vi "1 Channel N Samples - Manual Timestamps.vi"() -> ()   [LabVIEW 2026, in "synnax_lib.lvlib"]
uses:
  lvproj/lvlib/synnax_lib.lvlib
  lvproj/lvlib/typedefs/connection_config.ctl
  lvproj/lvlib/classes/Client/Private/synnax channel retrieve keys Single.vi
  lvproj/lvlib/classes/Writer/Private/synnax writer open Array.vi
  lvproj/lvlib/classes/Writer/Private/Writes/DBL/Write 1Ch NSamp (DBL).vi
  lvproj/lvlib/classes/Synnax Writer.lvclass
  lvproj/lvlib/classes/Client/Synnax Client.lvclass
panel:
  out "error out":errorcluster
  in  "Channel":string="my_f64_chan"
  in  "Stop":bool
  in  "Connection Config":T1={"host"="localhost", "port"=9090, "username"="synnax", "password"="seldon"}
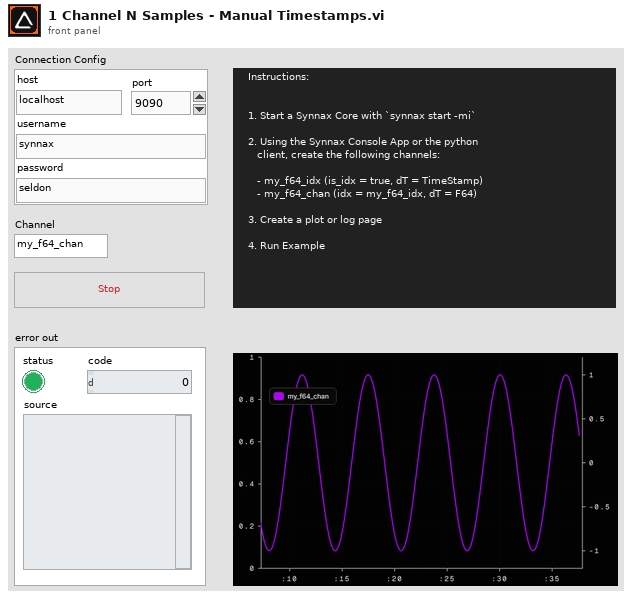
[diagram p1: front panel]
types:
  T1 = typedef "synnax_lib.lvlib/connection_config.ctl" = cluster{"host":string, "port":u16, "username":string, "password":string}
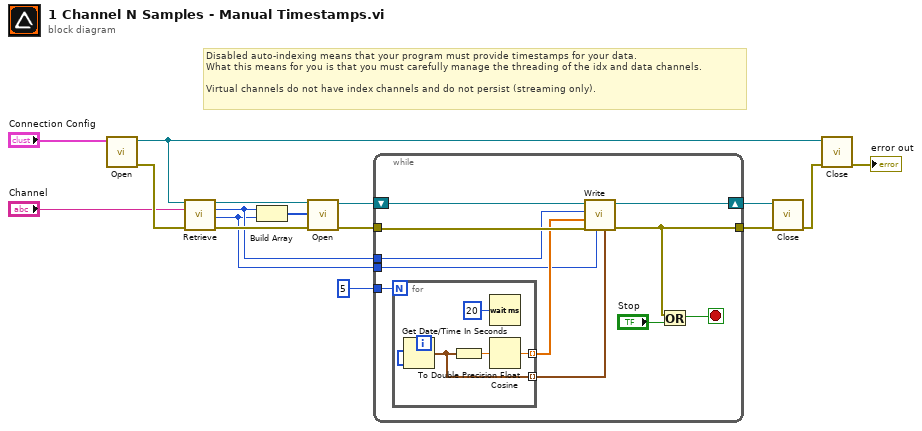
[diagram p0: block diagram]
diagram:
  # "Disabled auto-indexing means that your program must provide timestamps for your data.\nWhat this means for you is that you must carefully manage the threading of the idx and data channels.\n\nVirtual channels do not have index channels and do not persist (streaming only)."
  n1 = call "Open.vi"("Connection Config"="Connection Config") -> ("error out"=w11:errorcluster, "Synnax Client out"=w13:refnum<class "Synnax Client.lvclass">)  [unwired: 9 in]
  n2 = call-poly "Retrieve.vi"("Synnax Client in"=w13, "channel name"="Channel", "error in"=w11) -> ("Synnax Client out"=w7:refnum<class "Synnax Client.lvclass">, "channel key"=w4:u32, "index key"=w3:u32, "error out"=w15:errorcluster)  [unwired: 8 in, 1 out]
  n3 = Build Array(w4, w3) -> (w5:u32[])
  n4 = call-poly "Open.vi"("error in"=w15, "channels in"=w5, "Synnax Client in"=w7) -> ("error out"=w8:errorcluster, "writer out"=w10:refnum<class "Synnax Writer.lvclass">)  [unwired: 6 in, 1 out]
  n5 = while {
    shift-right: [w26] -> w9
    shift-left: w10 -> [w27]
    tunnel: w8 -> [w25]
    tunnel: [w17] -> w16
    tunnel: w3 -> [w22]
    tunnel: w4 -> [w20]
    tunnel: 5 -> [w19]
    stop <- w18 stop-if-true
    n6 = for {
      N: w19 -> [_]
      tunnel: [w31] -> w23 mode=indexing
      tunnel: [w29] -> w21 mode=indexing
      n7 = Get Date/Time In Seconds() -> (seconds since 1Jan1904=w29:timestamp)
      n8 = To Double Precision Float(number=w29) -> (double precision float=w30:dbl)
      n9 = Wait (ms)(milliseconds to wait=u32 20) -> ()  [unwired: 1 out]
      n10 = Cosine(x=w30) -> (cos(x)=w31:dbl)
    }
    n11 = call-poly "Write.vi"("timestamps"=w21, "index_channel"=w22, "error in"=w25, "data"=w23, "channel"=w20, "Writer"=w27) -> ("error out"=w17:errorcluster, "Writer Out"=w26:refnum<class "Synnax Writer.lvclass">)  [unwired: 4 in]
    n12 = Or(x=w17, y="Stop") -> (x .or. y?=w18:bool)
  }
  n13 = call "Close.vi"("error in"=w16, "writer"=w9) -> ("error out"=w12:errorcluster)  [unwired: 9 in]
  n14 = call "Close.vi"("error in"=w12, "Synnax Client in"=w13) -> ("error out"=→"error out":errorcluster)  [unwired: 9 in]
